vi "CODMn流程质控自动启动.vi"(0 "参数":T1={"是否启用仪器"=FALSE, "CODMn"={"启动测量模式"={"测量模式"=enum."水样测量"}, "确定按钮"=TRUE}, "启动模块"={"氨氮"=FALSE, "总磷"=FALSE, "总氮"=FALSE, "COD"=FALSE}, "常规启动"=FALSE, "直接启动"=FALSE}, 1 "CODMn量程切换":enum32{"H", "L", "AUTO"}(ring)=enum."AUTO") -> ()   [LabVIEW 2016, in "质控单元.lvlib"]
uses:
  PLC/PLC.lvlib
panel:
  out "枚举 2":enum16{"初始化", "采配水启动", "等待", "配水", "排水", "结束"}(ring)
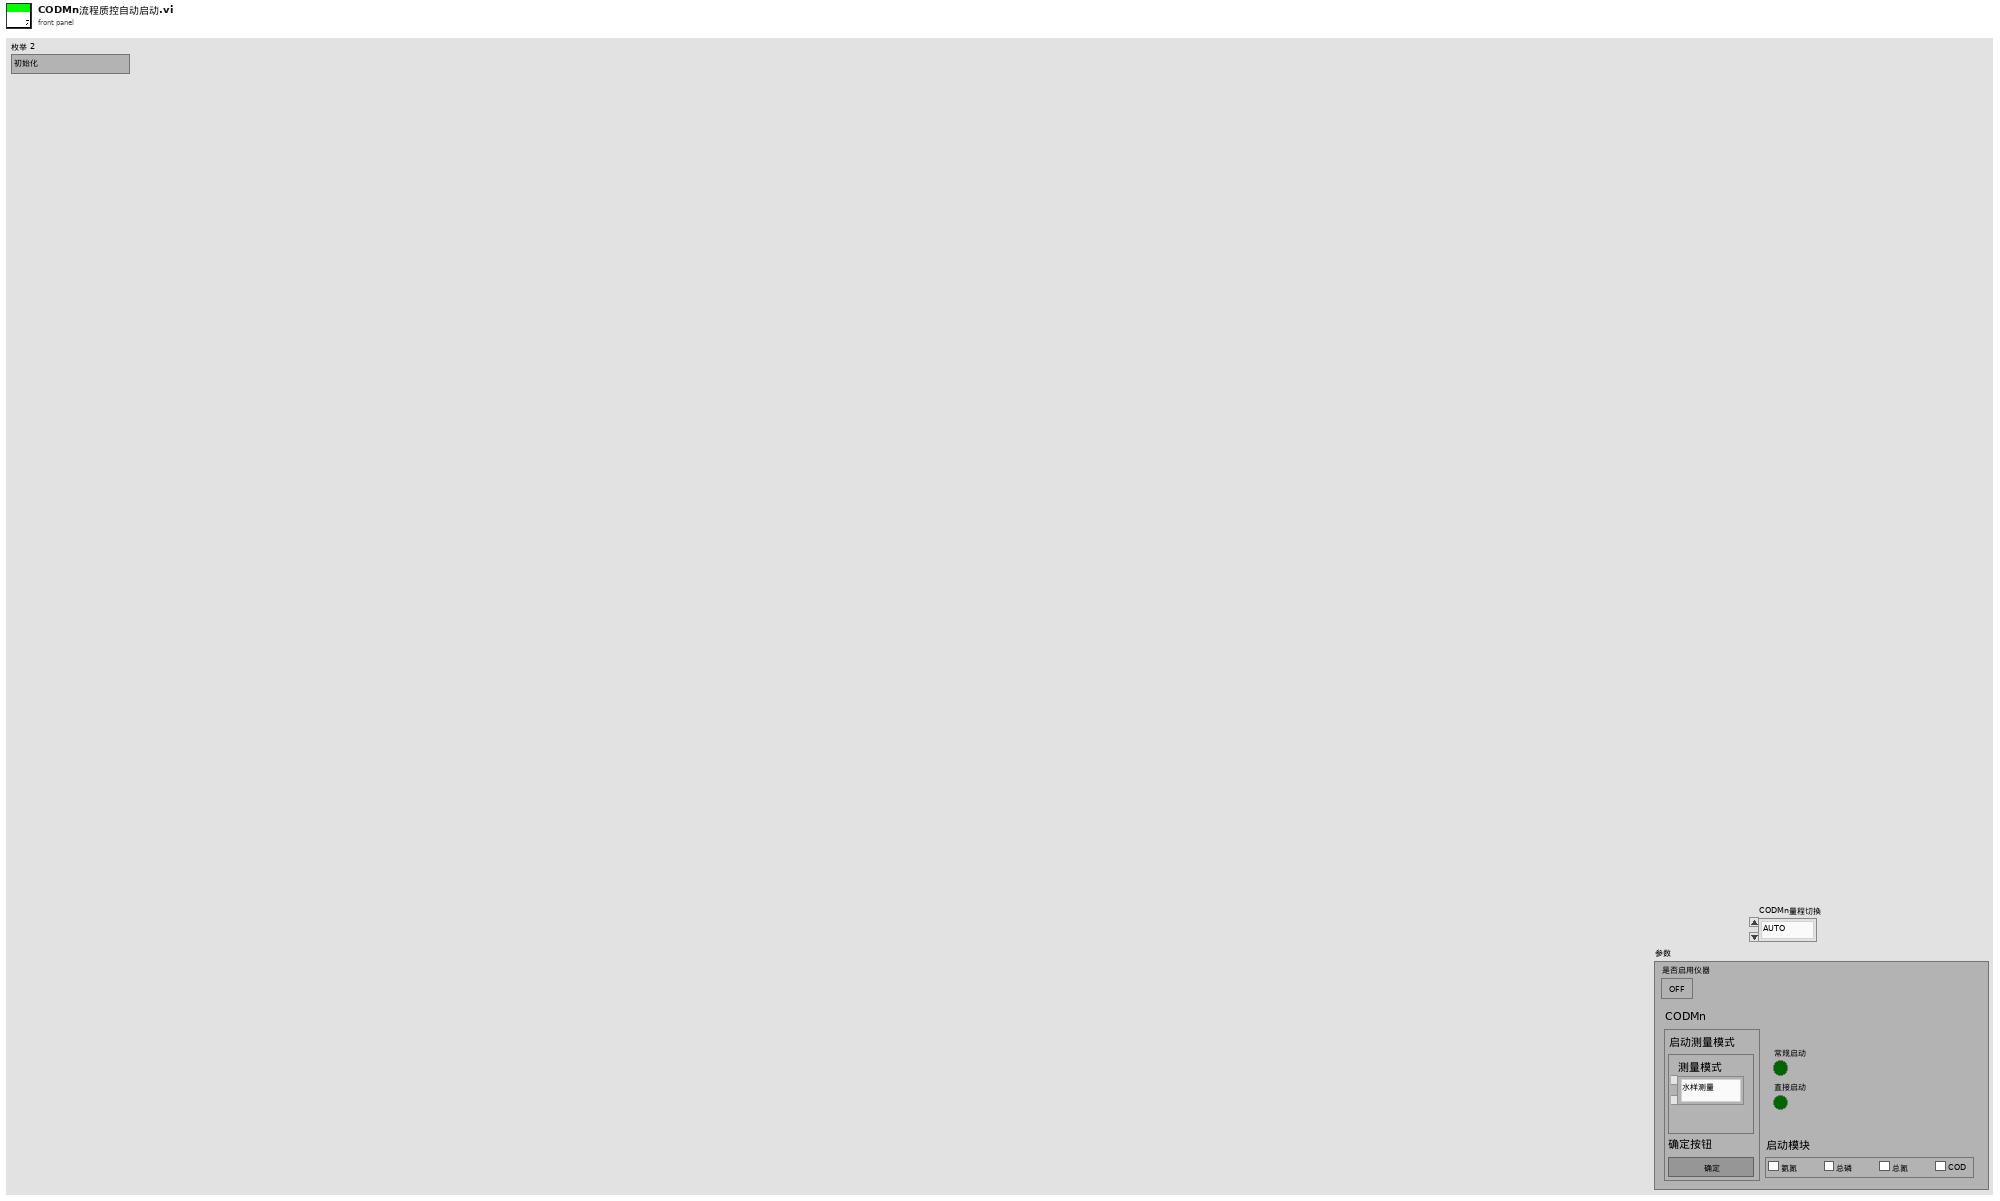
[diagram p1: front panel]
types:
  T1 = cluster{"是否启用仪器":bool, "CODMn":cluster{"启动测量模式":cluster{"测量模式":enum16{"水样测量", "标样核查", "加标回收", "平行样", "校零", "校标"}}, "确定按钮":bool}, "启动模块":cluster{"氨氮":bool, "总磷":bool, "总氮":bool, "COD":bool}, "常规启动":bool, "直接启动":bool}
  T2 = cluster{"R0":i16, "R1":i16, "R2":i16, "R3":i16, "R4":i16, "R5":i16, "R6":i16, "R7":i16, "R8":i16, "R9":i16, "R10":i16, "R11":i16, "R12":i16, "R13":i16, "R14":i16, "R15":i16, "R16":i16, "R17":i16, "R18":i16, "R19":i16, "R20":i16, "R21":i16, "R22":i16, "R23":i16, "R24":i16, "R25":i16, "R26":i16, "R27":i16, "R28":i16, "R29":i16, "R30":i16, "R31":i16, "R32":i16, "R33":i16, "R34":i16, "R35":i16, "R36":i16, "R37":i16, "R38":i16, "R39":i16, "R40":i16, "R41":i16, "R42":i16, "R43":i16, "R44":i16, "R45":i16, "R46":i16, "R47":i16, "R48":i16, "R49":i16, "R50":i16, "R51":i16, "R52":i16, "R53":i16, "R54":i16, "R55":i16}
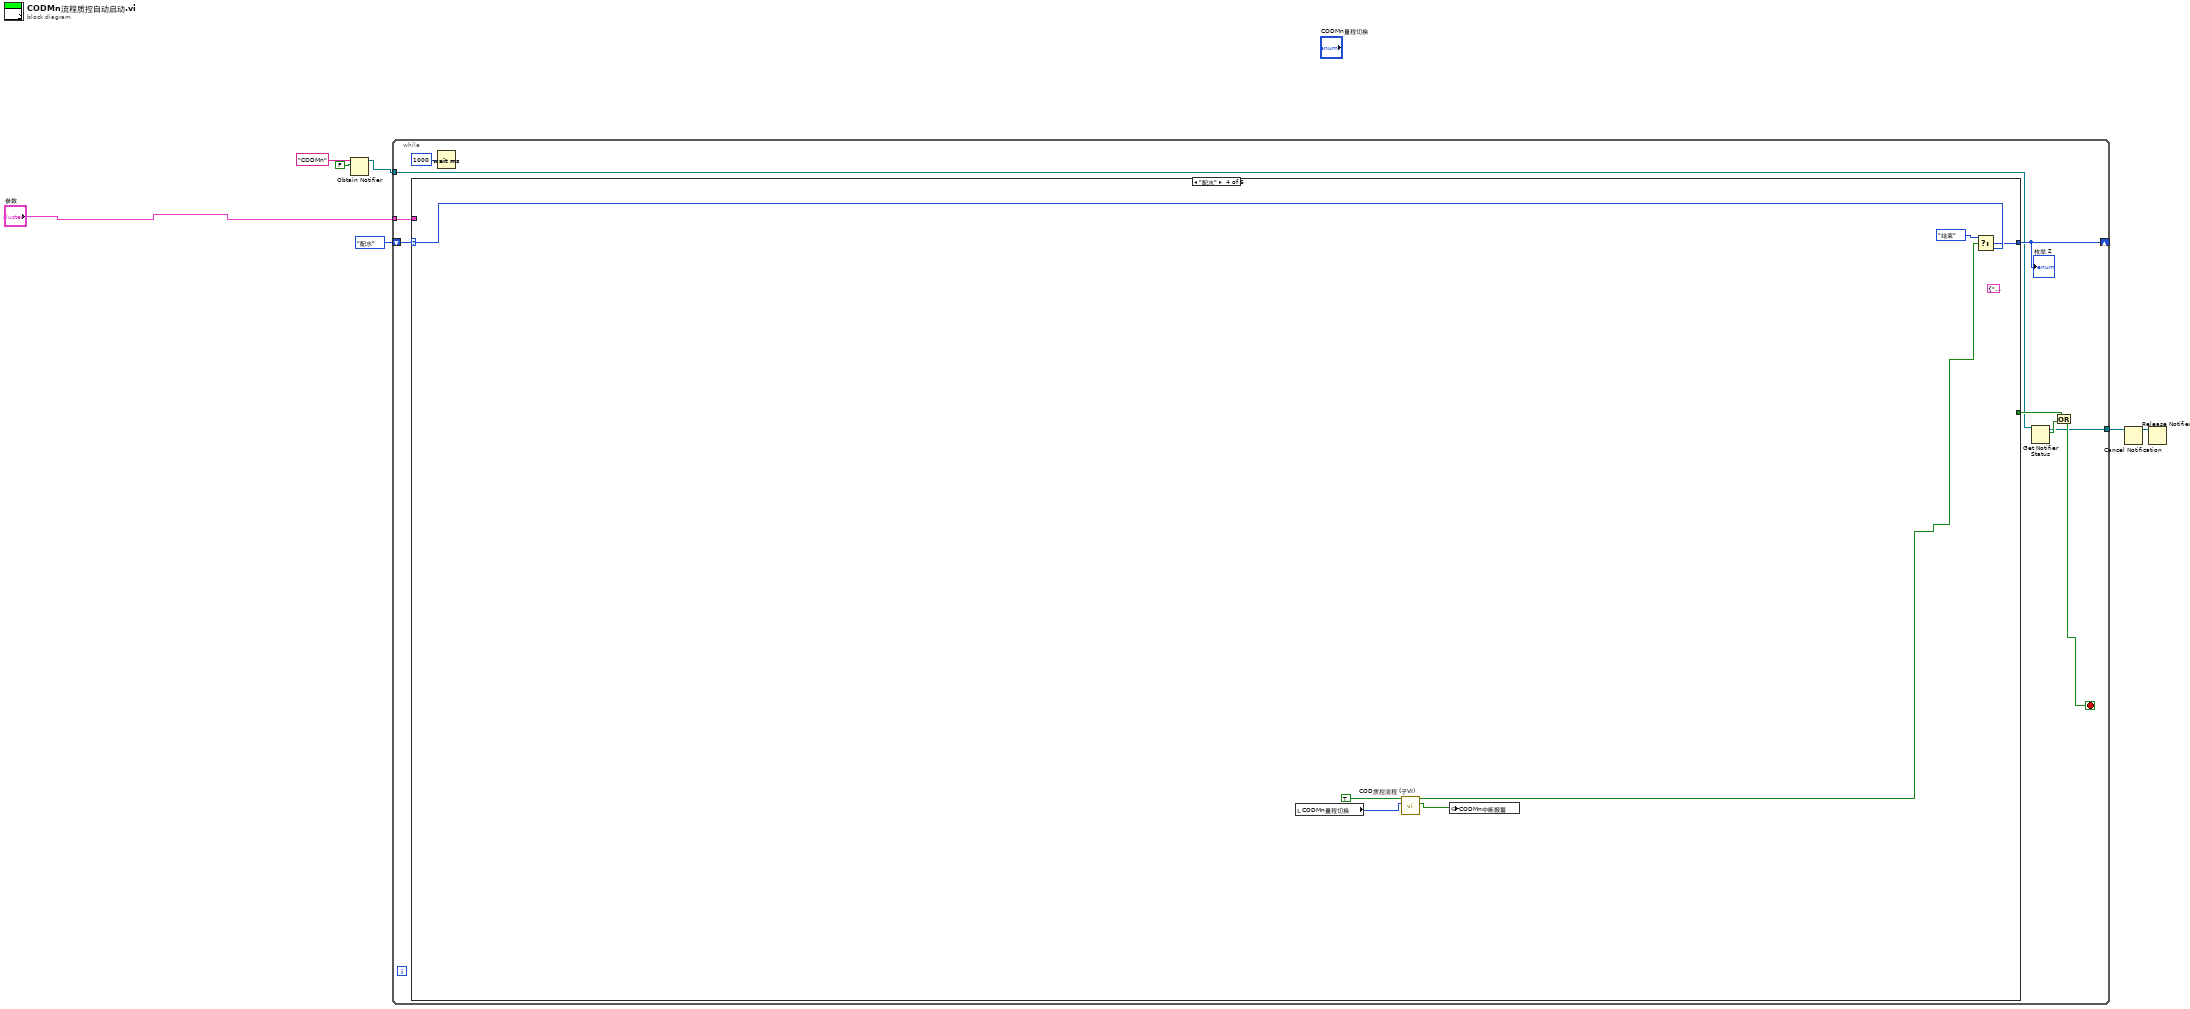
[diagram p0: block diagram]
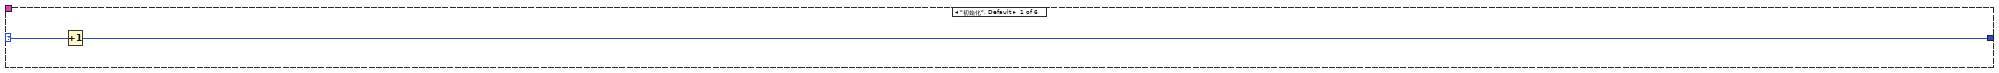
[diagram p2: hidden frame]
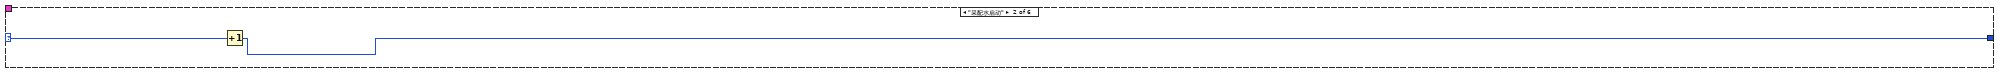
[diagram p3: hidden frame]
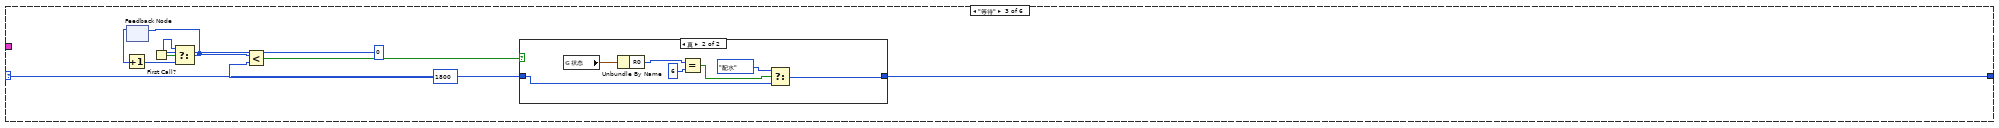
[diagram p4: hidden frame]
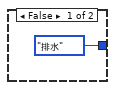
[diagram p5: hidden frame]
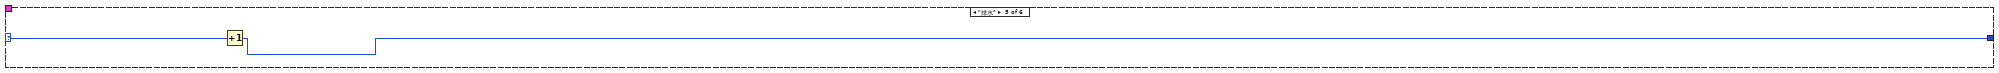
[diagram p6: hidden frame]
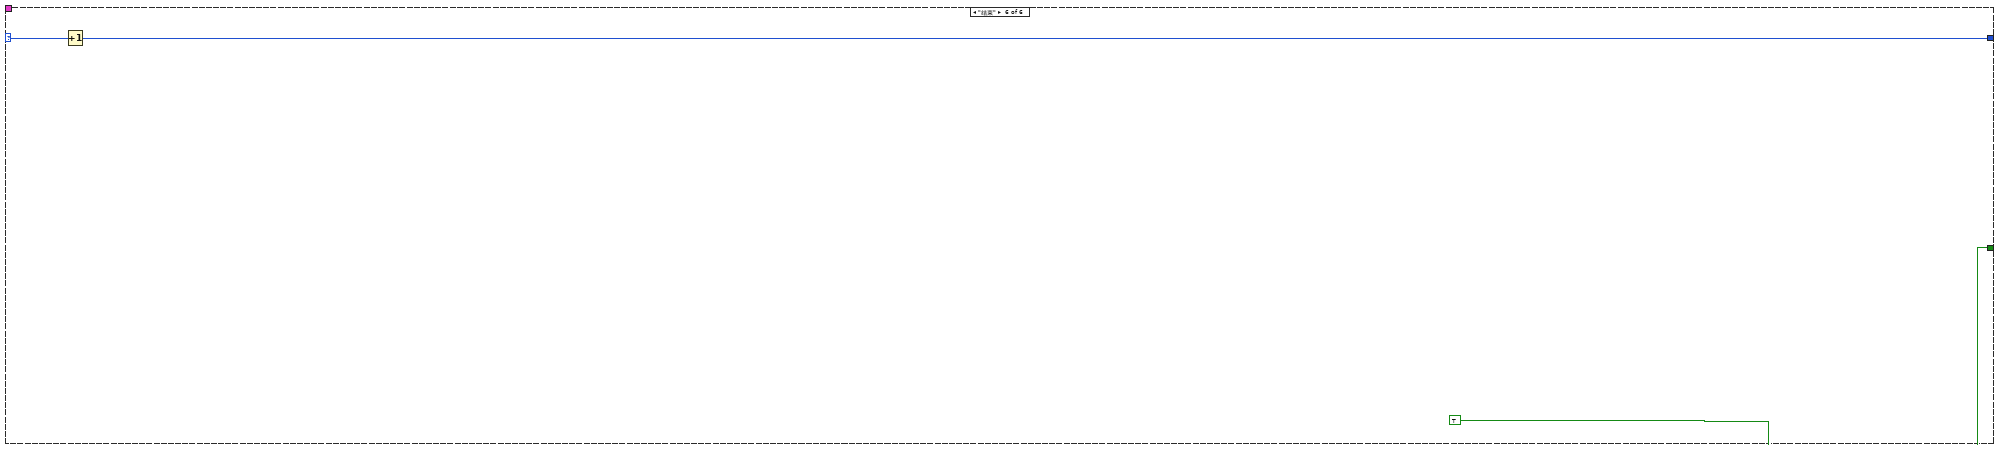
[diagram p7: hidden frame]
diagram:
  n1 = Obtain Notifier(name (unnamed)="CODMn" ("名称（未命名）"), notification data type=FALSE) -> (notifier out=w3:refnum<notifier>)  [unwired: 2 in, 2 out]
  n2 = while {
    shift-right: [w15] -> _
    shift-left: enum16{"初始化", "采配水启动", "等待", "配水", "排水", "结束"}."配水" ("枚举") -> [w16]
    tunnel: "参数" -> [w13]
    tunnel: w3 -> [w9]
    tunnel: [w8] -> w1
    stop <- w11 stop-if-true
    n3 = case shown="\"配水\"" w16 {
      selector: w16 -> [w18 w20 w27 w43 w46 w49]
      tunnel: [w17 w19 w26 w42 w45 w48] -> w15
      tunnel: [_ _ _ _ _ TRUE] -> w12
      tunnel: w13 -> [_ _ _ _ _ _]
      frame "初始化", Default {
        n4 = Increment(x=w18) -> (x+1=w17:enum16{"初始化", "采配水启动", "等待", "配水", "排水", "结束"})
      }
      frame "采配水启动" {
        n5 = Increment(x=w20) -> (x+1=w19:enum16{"初始化", "采配水启动", "等待", "配水", "排水", "结束"})
      }
      frame "等待" {
        n6 = feedback #1() -> (w23:i32)  [unwired: 1 in]
        n7 = Increment(x=w23) -> (x+1=w22:i32)
        n8 = First Call?() -> (First Call?: T/F=w24:bool)
        n9 = Select(t=0, s=w24, f=w22) -> (s? t:f=w21:i32)
        n10 = feedback-in #1(w21) -> ()
        n11 = Less?(x=w21, y=1800) -> (x < y?=w28:bool)
        n12 = case shown="真" w28 {
          tunnel: w27 -> [_ w32]
          tunnel: [enum16{"初始化", "采配水启动", "等待", "配水", "排水", "结束"}."排水" ("枚举") w31] -> w26
          frame False {
          }
          frame True {
            n13 = global read "采配水全局变量.vi" "状态"() -> (w37:T2)
            n14 = Unbundle By Name(w37) -> ("R0"=w36:i16)
            n15 = Equal?(x=w36, y=i16 6) -> (x = y?=w34:bool)
            n16 = Select(t=enum16{"初始化", "采配水启动", "等待", "配水", "排水", "结束"}."配水" ("枚举"), s=w34, f=w32) -> (s? t:f=w31:enum16{"初始化", "采配水启动", "等待", "配水", "排水", "结束"})
          }
        }
      }
      frame "配水" {
        (unwired) cluster{"命令":string, "data":variant} {"命令"="启动", "data"=variant(cluster{"站号":u16, "控制命令输出":u16[]} {"站号"=1, "控制命令输出"=[256, 0]})} ("元素")
        n17 = local read "CODMn量程切换"() -> (w40:enum32{"H", "L", "AUTO"})
        n18 = call "COD质控流程 (子VI).vi"("CODMn量程切换"=w40, "COD"=TRUE) -> ("CODMn中断报警"=w38:bool, "布尔"=w39:bool)  [unwired: 8 in]
        n19 = global write "质控中断报警全局.vi" "CODMn中断报警"(w38) -> ()
        n20 = Select(t=enum16{"初始化", "采配水启动", "等待", "配水", "排水", "结束"}."结束" ("枚举"), s=w39, f=w43) -> (s? t:f=w42:enum16{"初始化", "采配水启动", "等待", "配水", "排水", "结束"})
      }
      frame "排水" {
        n21 = Increment(x=w46) -> (x+1=w45:enum16{"初始化", "采配水启动", "等待", "配水", "排水", "结束"})
      }
      frame "结束" {
        n22 = Increment(x=w49) -> (x+1=w48:enum16{"初始化", "采配水启动", "等待", "配水", "排水", "结束"})
      }
    }
    "枚举 2" <- w15
    n23 = Wait (ms)(milliseconds to wait=u32 1000 ("等待时间（毫秒）")) -> ()  [unwired: 1 out]
    n24 = Get Notifier Status(notifier=w9) -> (notifier out=w8:refnum<notifier>, current notification=w10:bool)  [unwired: 1 in, 3 out]
    n25 = Or(x=w12, y=w10) -> (x .or. y?=w11:bool)
  }
  n26 = Cancel Notification(0:w1) -> (8:w2:refnum<notifier>)  [unwired: 1 in, 2 out]
  n27 = Release Notifier(notifier=w2) -> ()  [unwired: 2 in, 3 out]
